vi "meTEC Control Software.vi"() -> ()   [LabVIEW 2019]
doc: "This is the vi discription of the Top Level VI"
uses:
  LV Source/[meerstetter engineering TE Cooling]/TypeDefs/meTEC_ID 50000_Live Enable.ctl
  LV Source/[meerstetter engineering TE Cooling]/TypeDefs/meTEC_ID 2000_Input Selection.ctl
  LV Source/[meerstetter engineering TE Cooling]/TypeDefs/meTEC_ID 50011_Object Target Temperature Source Selection.ctl
  LV Source/[meerstetter engineering TE Cooling]/TypeDefs/meTEC_ID 104_Device Status.ctl
  LV Source/[meerstetter engineering TE Cooling]/TypeDefs/meTEC_ID 1200_Temperature is Stable.ctl
  LV Source/Type Definitions/Main Loop Queue Data.ctl
  LV Source/Type Definitions/Main Loop States.ctl
  LV Source/Variables/FGVs/Type Defs/FGV_Operations.ctl
  <vilib>/Utility/error.llb/DialogType.ctl
  LV Source/Variables/Globals/Global_Initialized.vi
  LV Source/Variables/Globals/Global_TEC Monitor Loop_Status.vi
  LV Source/Variables/Globals/Global_Quit.vi
panel:
  out "Control Suite Status":string
  in  "Tab Control_General":T1(tab)
  out "meTEC_Device Type":string caption="Device Type"
  out "meTEC_CH1_Device Status":T2=1 caption="Device Status" items=["Initializing", "Ready", "Run", "Error", "Bootloader", "Reset in Progress"]
  out "meTEC_CH1_Temperature Stability":T3=1 caption="Temperature Stabilty" items=["Temperature regulation is not active", "Is not stable", "Is stable"]
  out "meTEC_CH1_Object Temperature [°C]":dbl caption="Object Temperature [°C]" format="%.3f"
  out "meTEC_CH1_Sink Temperature [°C]":dbl caption="Sink Temperature [°C]" format="%.3f"
  out "meTEC_CH1_Act. Output Voltage [V]":dbl caption="Act. Output Voltage [V]" format="%.3f"
  out "meTEC_CH1_Act. Output Current [A]":dbl caption="Act. Output Current [A]" format="%.3f"
  out "meTEC_Hardware Version":string caption="Hardware Version"
  out "meTEC_Firmware Version":string caption="Firmware Version"
  out "meTEC_Serial No.":i32 caption="Serial No."
  out "meTEC_CH1_Error No.":i32 caption="Error No."
  out "meTEC_CH1_Error Instance":i32 caption="Error Instance"
  out "meTEC_CH1_Error Parameter":i32 caption="Error Parameter"
  out "meTEC_CH2_Temperature Stability":T3=1 caption="Temperature Stabilty" items=["Temperature regulation is not active", "Is not stable", "Is stable"]
  out "meTEC_CH2_Act. Output Current [A]":dbl caption="Act. Output Current [A]" format="%.3f"
  out "meTEC_CH2_Act. Output Voltage [V]":dbl caption="Act. Output Voltage [V]" format="%.3f"
  out "meTEC_CH2_Object Temperature [°C]":dbl caption="Object Temperature [°C]" format="%.3f"
  out "meTEC_CH2_Sink Temperature [°C]":dbl caption="Sink Temperature [°C]" format="%.3f"
  out "Monitor Chart_CH2":dbl[](graph)
  out "Monitor Chart_CH1":dbl[](graph)
  out "Loop Rate [ms]":u32 caption="Update Rate [ms]"
  in  "meTEC_Reset Device":bool caption="Reset Device"
  in  "meTEC_CH1_Live Enable (ID 50000)":T4 caption="Live Enable (ID 50000)" items=["Disabled (Reset State)", "Enabled"]
  in  "meTEC_CH1_Input Selection (ID 2000)":T5=2 caption="Input  Selection (ID 2000)" items=["Static Current / Voltage", "Live Current / Voltage", "Temperature Controller"]
  in  "meTEC_CH1_Object Target Temp. Source Selection (ID 50011)":T6 caption="Object Target Temperature Source Selection (ID 50011)" items=["Parameter ID 3000 (Reset State)", "Parameter ID 50012"]
  in  "meTEC_CH1_Object Target Temperature (ID 3000 / 50012) [°C]":dbl=23.0 caption="Object Target Temperature (ID 3000 / 50012) [°C]" min=-273.0 max=1000.0 step=0.001 format="%#.3f"
  in  "meTEC_CH1_Live Set Current (ID 50001) [A]":dbl caption="Live Set Current (ID 50001) [A]" min=-16.0 max=16.0 step=0.001 format="%#.3f"
  in  "meTEC_CH2_Object Target Temperature (ID 3000 / 50012) [°C]":dbl=23.0 caption="Object Target Temperature (ID 3000) [°C]" min=-273.0 max=1000.0 step=0.001 format="%#.3f"
  in  "meTEC_CH2_Live Set Current (ID 50001) [A]":dbl caption="Live Set Current (ID 50001) [A]" min=-16.0 max=16.0 step=0.001 format="%#.3f"
  in  "meTEC_CH1_Live Set Voltage (ID 50002) [V]":dbl caption="Live Set Voltage (ID 50002) [V]" min=0.0 max=30.0 step=0.001 format="%#.3f"
  in  "meTEC_CH2_Live Set Voltage (ID 50002) [V]":dbl caption="Live Set Voltage (ID 50002) [V]" min=0.0 max=30.0 step=0.001 format="%#.3f"
  in  "meTEC_CH2_Object Target Temp. Source Selection (ID 50011)":T6 caption="Object Target Temperature Source Selection (ID 50011)" items=["Parameter ID 3000 (Reset State)", "Parameter ID 50012"]
  in  "meTEC_CH2_Input Selection (ID 2000)":T5=2 caption="Input  Selection (ID 2000)" items=["Static Current / Voltage", "Live Current / Voltage", "Temperature Controller"]
  in  "meTEC_CH2_Live Enable (ID 50000)":T4 caption="Live Enable" items=["Disabled (Reset State)", "Enabled"]
  in  "meTEC_Initialize Device":bool caption="Initialize Device"
  in  "meTEC_Perform Test":bool caption="Execute Test"
  out "Error History Table":string[][](table) caption="Error History"
  in  "Filepath Error Log File":path=path "C:/Error Data"
  in  "Show Pop-Ups for Error Messages?":bool
  in  "meTEC_Error Test 1_ID100_Device Type":bool caption="Error Test"
  # "Channel 1"
  # "Channel 2"
  # "General"
  # "Channel 1"
  # "Channel 2"
  # "Please set \"CH1 Output Stage Enable\" to\n\"Live ON/OFF\" in meerstetter engineering\nservice software.\n\nAfter that you can switch the TE controller\nON / OFF by changing the \"Live Enable\"\nsetting in this LabVIEW example."
  # "Please set \"CH2 Output Stage Enable\" to\n\"Live ON/OFF\" in meerstetter engineering\nservice software.\n\nAfter that you can switch the TE controller\nON / OFF by changing the \"Live Enable\"\nsetting in this LabVIEW example."
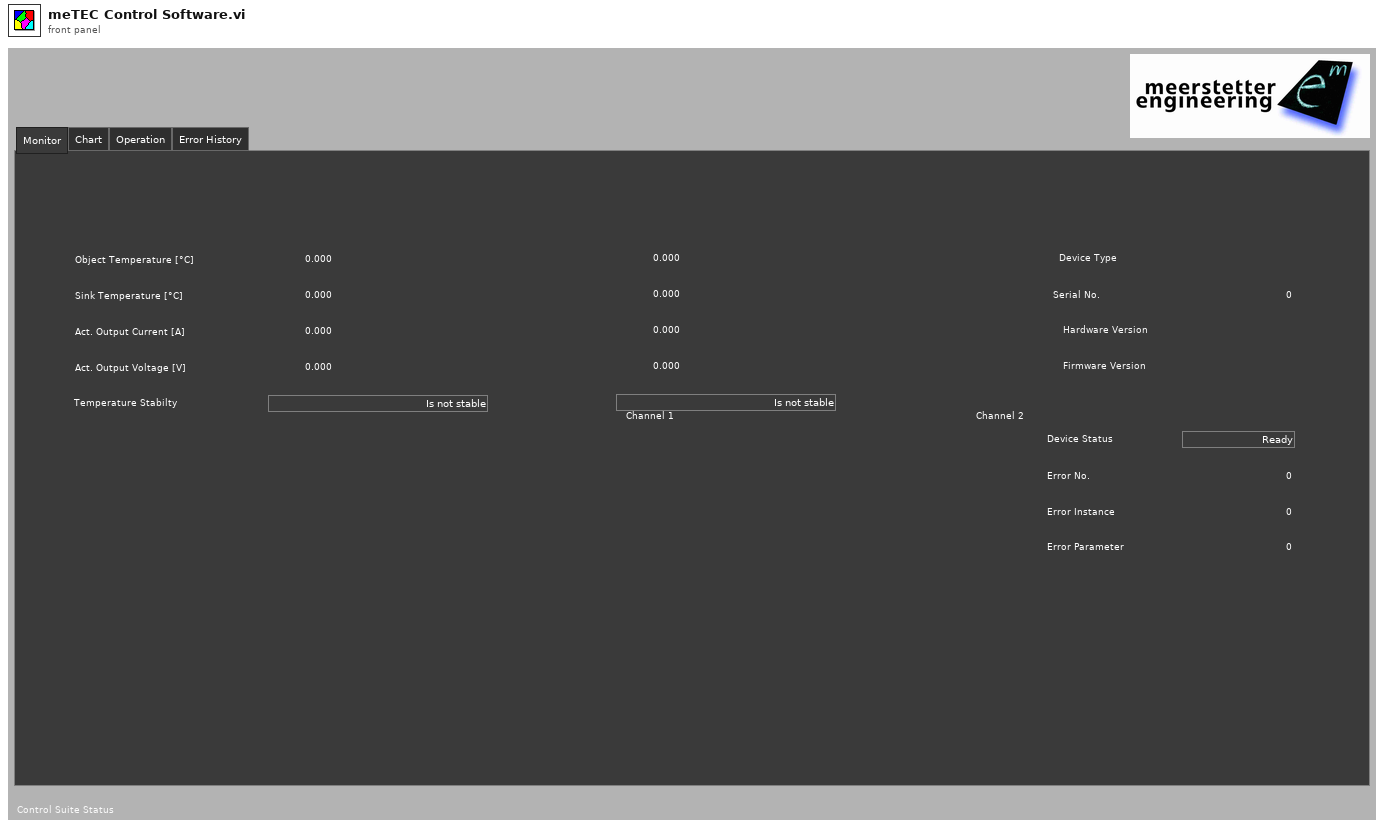
[diagram p1: front panel]
types:
  T1 = enum32{"Monitor", "Chart", "Operation", "Error History"}
  T2 = typedef "meTEC_ID 104_Device Status.ctl" = i32
  T3 = typedef "meTEC_ID 1200_Temperature is Stable.ctl" = i32
  T4 = typedef "meTEC_ID 50000_Live Enable.ctl" = i32
  T5 = typedef "meTEC_ID 2000_Input Selection.ctl" = i32
  T6 = typedef "meTEC_ID 50011_Object Target Temperature Source Selection.ctl" = i32
  T7 = typedef "Main Loop States.ctl" = enum16{"  -----  Core  -----  ", "Blank", "Idle", "Initialize", "Shutdown", "Error", "  ----- meerstetter TEC Functions -----  ", "TE Controller"}
  T8 = typedef "Main Loop Queue Data.ctl" = cluster{"Parameter":string, "Variant":variant, "Main Loop States":T7}
  T9 = enum32{"invalid app kind", "Development System", "Run Time System", "Student Edition", "Embedded LabVIEW", "Evaluation", "Custom"}
  T10 = typedef "FGV_Operations.ctl" = enum16{"Read", "Write"}
  T11 = typedef "FGV_TE Controller.ctl" = cluster{"SVs":cluster{"Unused":dbl}, "PVs":cluster{"FW & HW Versions":cluster{"Device Type [I32]":i32, "Device Type [String]":string, "Firmware Version [I32]":i32, "Firmware Version [String]":string, "Hardware Version [I32]":i32, "Hardware Version [String]":string, "Serial No.":i32}, "TEC Configuration":T12, "Object Target Temperature Source_CH1":u8, "Object Target Temperature Source_CH2":u8}, "Front Panel References":T13}
  T12 = typedef "meTEC_Configuration.ctl" = cluster{"VISA resource name":refnum<visa-resource-name>, "Device Address":u16}
  T13 = typedef "FGV_Front Panel References.ctl" = cluster{"Main Loop Queue":refnum<queue>, "meTEC_Device Type":refnum<vi>, "meTEC_Serial No.":refnum<vi>, "meTEC_Hardware Version":refnum<vi>, "meTEC_Firmware Version":refnum<vi>, "meTEC_CH1_Object Target Temperature (ID 3000 / 50012) [°C]":refnum<vi>, "meTEC_CH1_Live Set Current (ID 50001) [A]":refnum<vi>, "meTEC_CH1_Live Set Voltage (ID 50002) [V]":refnum<vi>, "meTEC_CH1_Live Enable (ID 50000)":refnum<vi>, "meTEC_CH1_Input Selection (ID 2000)":refnum<vi>, "meTEC_CH1_Object Target Temp. Source Sel. (ID 50011)":refnum<vi>, "meTEC_CH2_Object Target Temperature (ID 3000 / 50012) [°C]":refnum<vi>, "meTEC_CH2_Live Set Current (ID 50001) [A]":refnum<vi>, "meTEC_CH2_Live Set Voltage (ID 50002) [V]":refnum<vi>, "meTEC_CH2_Live Enable (ID 50000)":refnum<vi>, "meTEC_CH2_Input Selection (ID 2000)":refnum<vi>, "meTEC_CH2_Object Target Temp. Source Sel. (ID 50011)":refnum<vi>, "meTEC_CH2_Object Temperature [°C]":refnum<vi>, "meTEC_CH2_Sink Temperature [°C]":refnum<vi>, "meTEC_CH2_Act. Output Current [A]":refnum<vi>, "meTEC_CH2_Act. Output Voltage [V]":refnum<vi>, "meTEC_CH2_Temperature Stability":refnum<vi>, "Monitor Chart_CH2":refnum<vi>, "meTEC_Initialize Device":refnum<vi>}
  T14 = typedef "DialogType.ctl" = u16
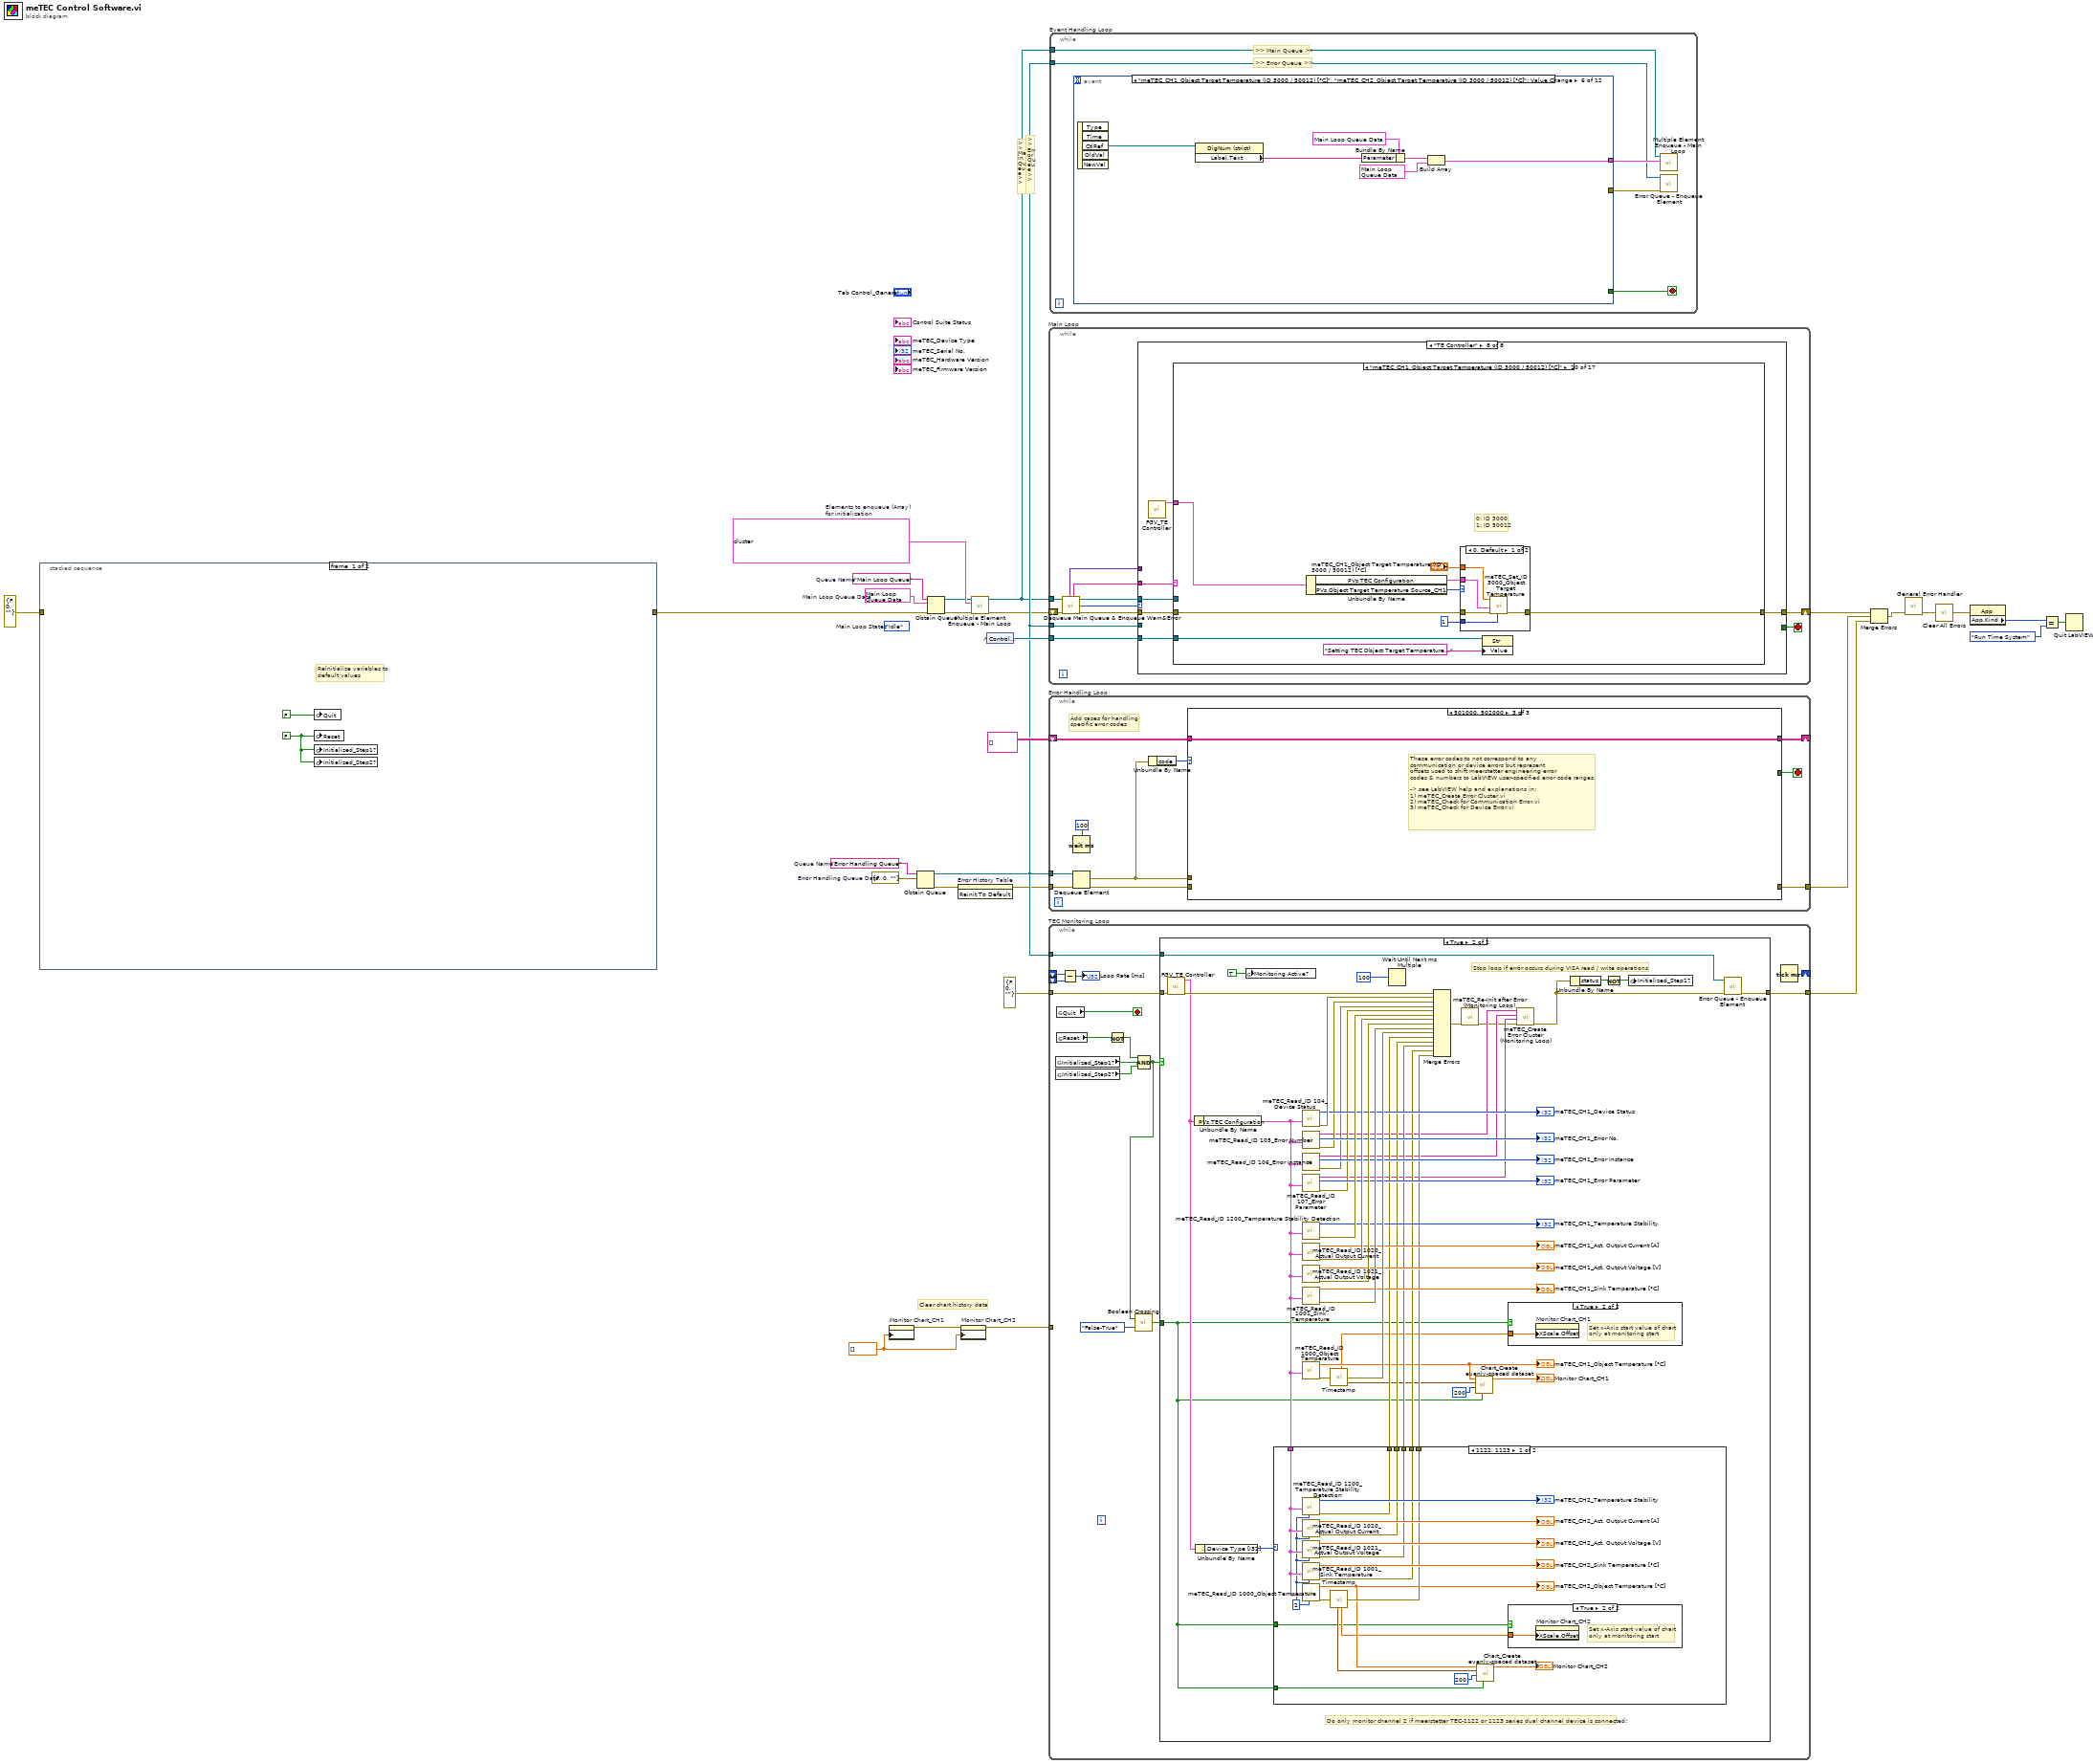
[diagram p0: block diagram]
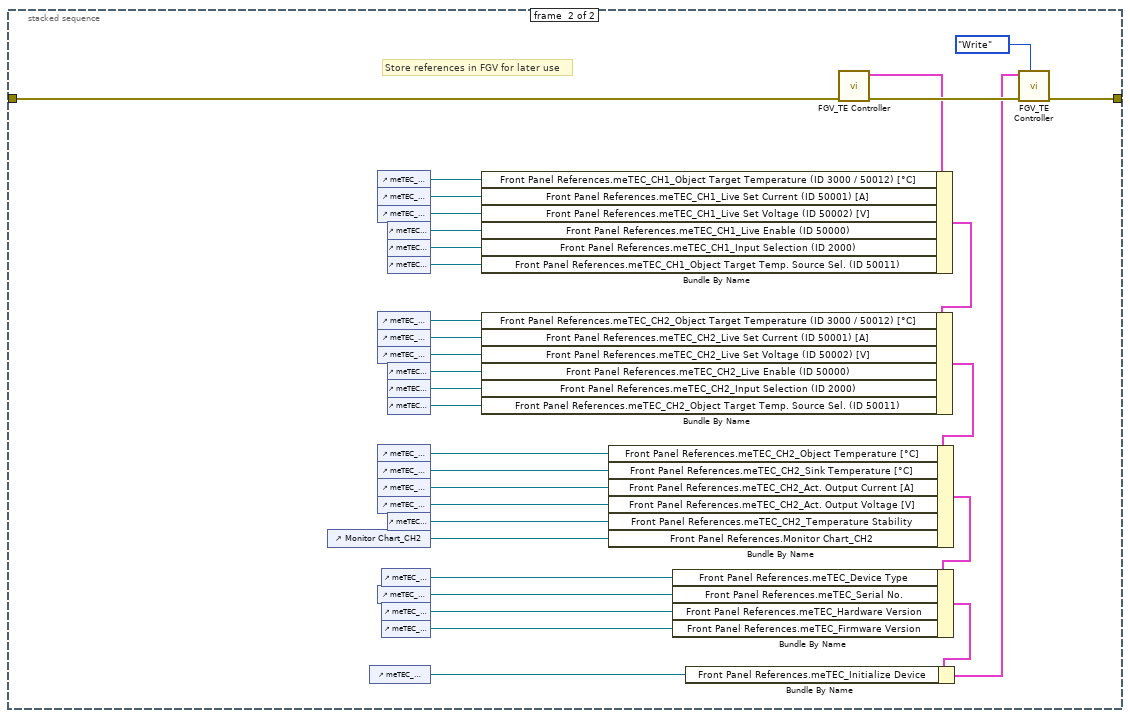
[diagram p2: hidden frame]
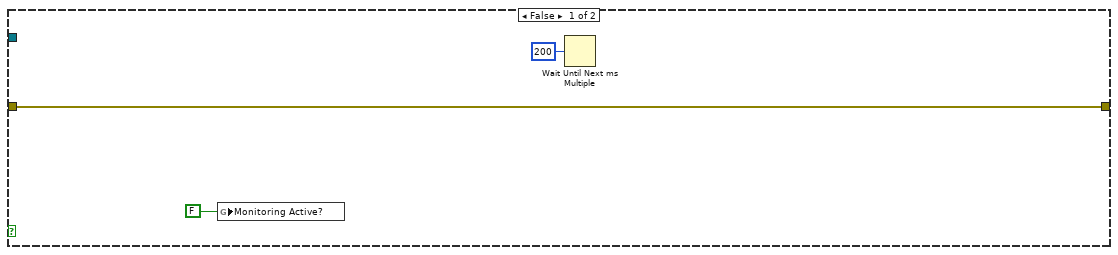
[diagram p3: hidden frame]
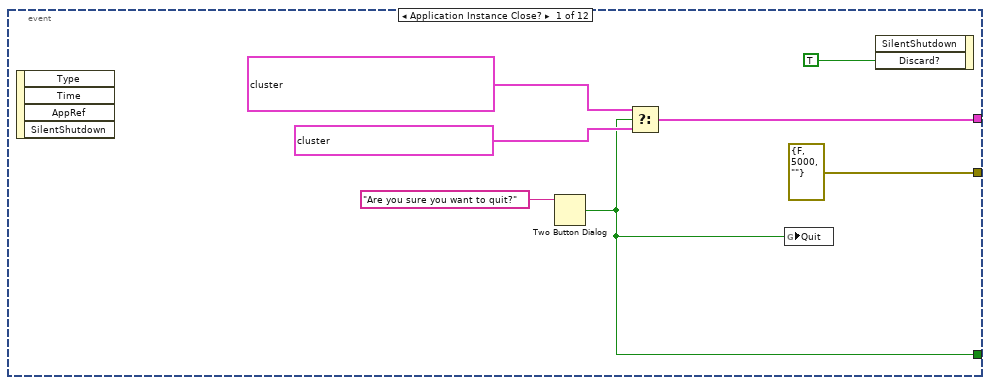
[diagram p7: hidden frame]
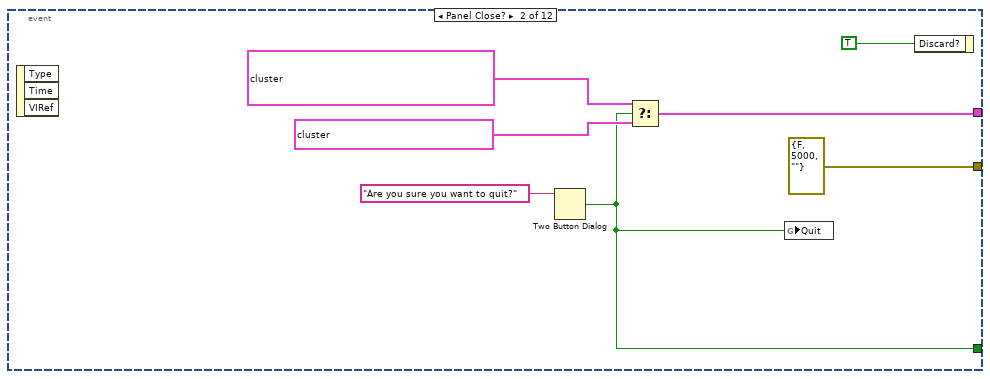
[diagram p8: hidden frame]
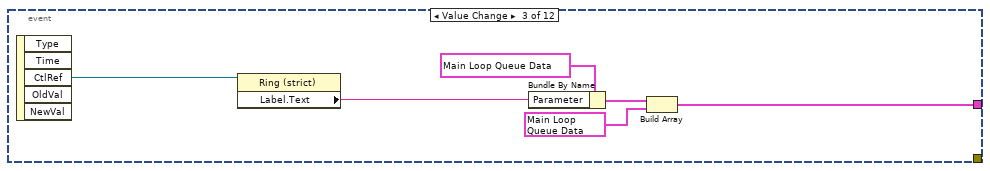
[diagram p9: hidden frame]
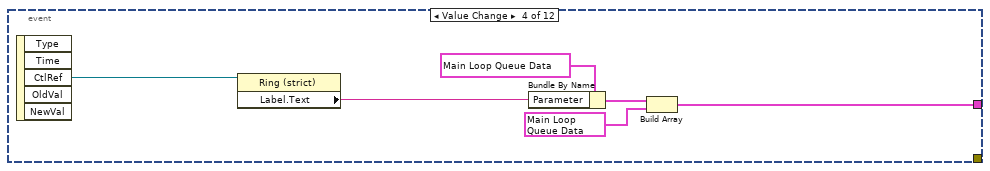
[diagram p10: hidden frame]
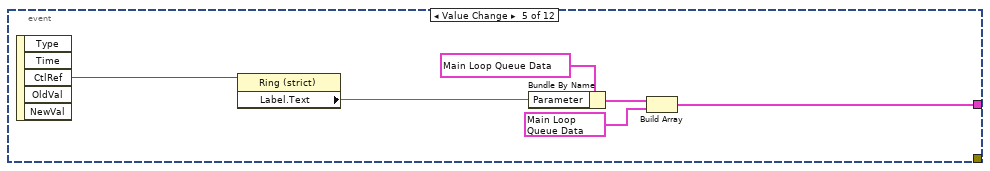
[diagram p11: hidden frame]
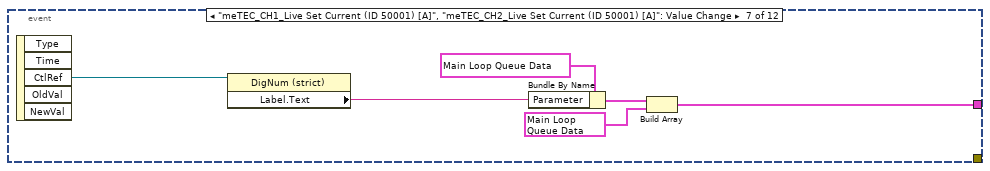
[diagram p12: hidden frame]
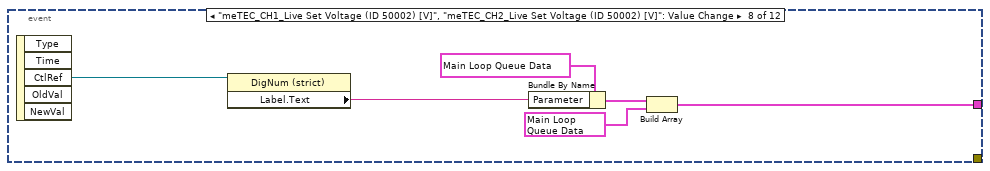
[diagram p13: hidden frame]
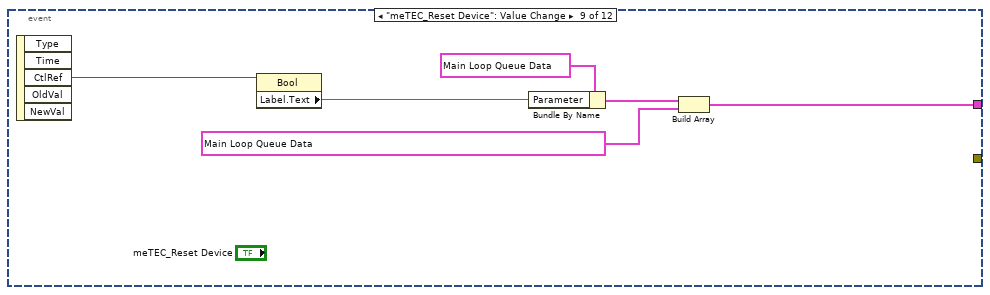
[diagram p14: hidden frame]
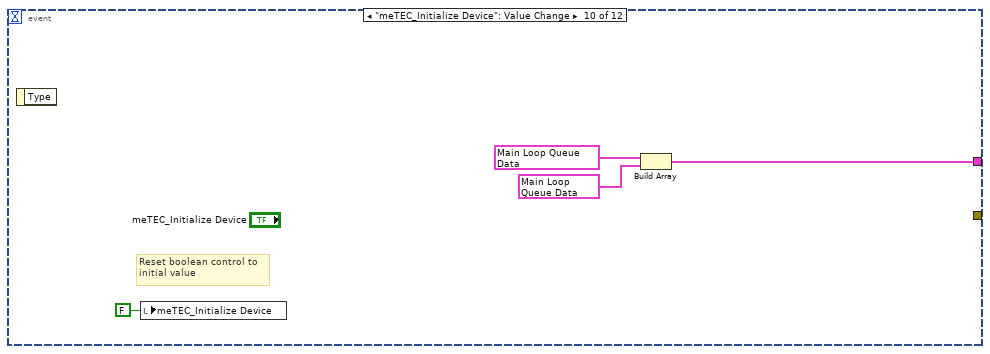
[diagram p15: hidden frame]
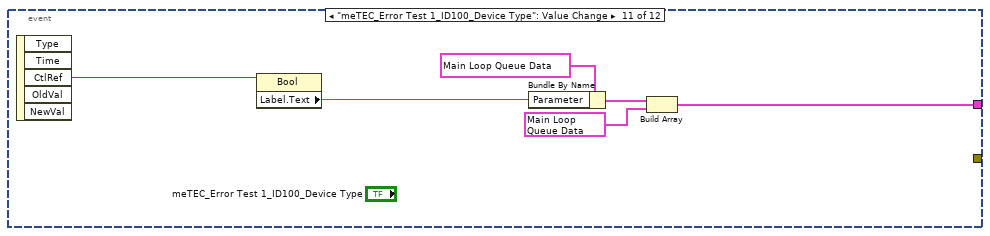
[diagram p16: hidden frame]
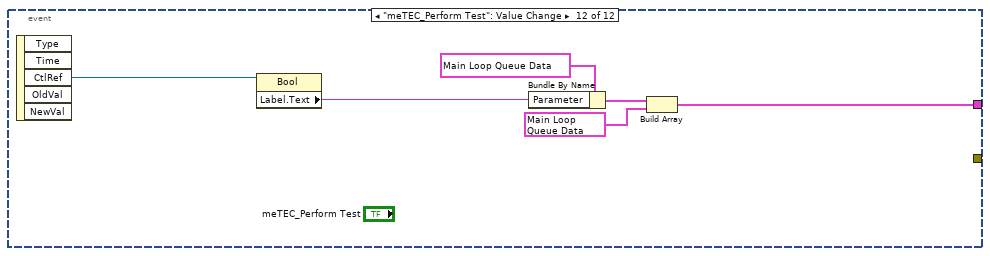
[diagram p17: hidden frame]
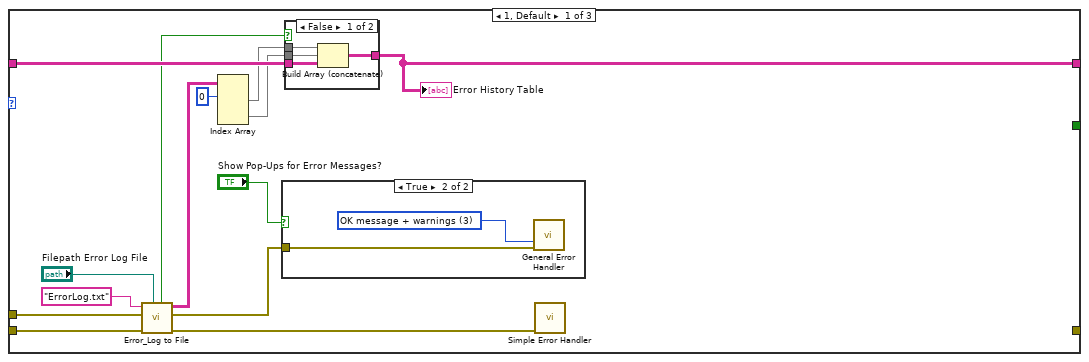
[diagram p18: hidden frame]
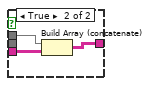
[diagram p19: hidden frame]
diagram:
  w7 = dbl[] [] ("History Data")
  (unwired) Main_Loop_States."Idle"  # Main Loop States
  w19 = T8 {"Parameter"="", "Variant"=variant, "Main Loop States"=enum."Idle"}  # Main Loop Queue Data
  w24 = errorcluster {"status"=FALSE, "code"=0, "source"=""}  # Error Handling Queue Data
  w25 = "Error Handling Queue"  # Queue Name
  w26 = "Main Loop Queue"  # Queue Name
  w18 = T8[] [{"Parameter"="", "Variant"=variant, "Main Loop States"=enum."Initialize"}, {"Parameter"="", "Variant"=variant, "Main Loop States"=enum."Idle"}]  # Elements to enqueue (Array) for initialization
  # "Clear chart history data"
  # ">> Error Queue >>"
  # ">> Main Queue >>"
  n1 = stacked-sequence {
    tunnel: [_ w63] -> w11
    tunnel: errorcluster {"status"=FALSE, "code"=0, "source"=""} ("error out") -> [_ w64]
    frame #0 {
      w31 = FALSE ("Error")
      # "Reinitialize variables to\ndefault values"
      n2 = global write "Global_Quit.vi" "Quit"(FALSE ("Quit")) -> ()
      n3 = global write "Global_TEC Monitor Loop_Status.vi" "Reset"(w31) -> ()
      n4 = global write "Global_Initialized.vi" "Initialized_Step1?"(w31) -> ()
      n5 = global write "Global_Initialized.vi" "Initialized_Step2?"(w31) -> ()
    }
    frame #1 {
      # "Store references in FGV for later use"
      n6 = control-ref of="Monitor Chart_CH2"() -> (w43:refnum<vi>)
      n7 = control-ref of="meTEC_Initialize Device"() -> (w38:refnum<vi>)
      n8 = control-ref of="meTEC_CH1_Object Target Temperature (ID 3000 / 50012) [°C]"() -> (w46:refnum<vi>)
      n9 = control-ref of="meTEC_CH1_Live Set Current (ID 50001) [A]"() -> (w44:refnum<vi>)
      n10 = control-ref of="meTEC_CH1_Live Set Voltage (ID 50002) [V]"() -> (w45:refnum<vi>)
      n11 = control-ref of="meTEC_CH2_Object Target Temperature (ID 3000 / 50012) [°C]"() -> (w60:refnum<vi>)
      n12 = control-ref of="meTEC_CH2_Live Set Current (ID 50001) [A]"() -> (w55:refnum<vi>)
      n13 = control-ref of="meTEC_CH2_Live Set Voltage (ID 50002) [V]"() -> (w56:refnum<vi>)
      n14 = control-ref of="meTEC_CH2_Object Temperature [°C]"() -> (w53:refnum<vi>)
      n15 = control-ref of="meTEC_CH2_Sink Temperature [°C]"() -> (w49:refnum<vi>)
      n16 = control-ref of="meTEC_CH2_Act. Output Current [A]"() -> (w50:refnum<vi>)
      n17 = control-ref of="meTEC_CH2_Act. Output Voltage [V]"() -> (w51:refnum<vi>)
      n18 = control-ref of="meTEC_Serial No."() -> (w34:refnum<vi>)
      n19 = control-ref of="meTEC_Device Type"() -> (w35:refnum<vi>)
      n20 = control-ref of="meTEC_Hardware Version"() -> (w33:refnum<vi>)
      n21 = control-ref of="meTEC_Firmware Version"() -> (w32:refnum<vi>)
      n22 = control-ref of="meTEC_CH1_Live Enable (ID 50000)"() -> (w41:refnum<vi>)
      n23 = control-ref of="meTEC_CH1_Input Selection (ID 2000)"() -> (w40:refnum<vi>)
      n24 = control-ref of="meTEC_CH1_Object Target Temp. Source Selection (ID 50011)"() -> (w39:refnum<vi>)
      n25 = control-ref of="meTEC_CH2_Live Enable (ID 50000)"() -> (w57:refnum<vi>)
      n26 = control-ref of="meTEC_CH2_Input Selection (ID 2000)"() -> (w58:refnum<vi>)
      n27 = control-ref of="meTEC_CH2_Object Target Temp. Source Selection (ID 50011)"() -> (w59:refnum<vi>)
      n28 = control-ref of="meTEC_CH2_Temperature Stability"() -> (w52:refnum<vi>)
      n29 = call "FGV_TE Controller.vi"("error in (no error)"=w64) -> ("error out"=w62:errorcluster, "FGV_TEC_OUT"=w48:T11)  [unwired: 9 in]
      n30 = Bundle By Name(cluster=w48, "Front Panel References.meTEC_CH1_Object Target Temperature (ID 3000 / 50012) [°C]"=w46, "Front Panel References.meTEC_CH1_Live Set Current (ID 50001) [A]"=w44, "Front Panel References.meTEC_CH1_Live Set Voltage (ID 50002) [V]"=w45, "Front Panel References.meTEC_CH1_Live Enable (ID 50000)"=w41, "Front Panel References.meTEC_CH1_Input Selection (ID 2000)"=w40, "Front Panel References.meTEC_CH1_Object Target Temp. Source Sel. (ID 50011)"=w39) -> (w47:T11)
      n31 = Bundle By Name(cluster=w47, "Front Panel References.meTEC_CH2_Object Target Temperature (ID 3000 / 50012) [°C]"=w60, "Front Panel References.meTEC_CH2_Live Set Current (ID 50001) [A]"=w55, "Front Panel References.meTEC_CH2_Live Set Voltage (ID 50002) [V]"=w56, "Front Panel References.meTEC_CH2_Live Enable (ID 50000)"=w57, "Front Panel References.meTEC_CH2_Input Selection (ID 2000)"=w58, "Front Panel References.meTEC_CH2_Object Target Temp. Source Sel. (ID 50011)"=w59) -> (w54:T11)
      n32 = Bundle By Name(cluster=w54, "Front Panel References.meTEC_CH2_Object Temperature [°C]"=w53, "Front Panel References.meTEC_CH2_Sink Temperature [°C]"=w49, "Front Panel References.meTEC_CH2_Act. Output Current [A]"=w50, "Front Panel References.meTEC_CH2_Act. Output Voltage [V]"=w51, "Front Panel References.meTEC_CH2_Temperature Stability"=w52, "Front Panel References.Monitor Chart_CH2"=w43) -> (w37:T11)
      n33 = Bundle By Name(cluster=w37, "Front Panel References.meTEC_Device Type"=w35, "Front Panel References.meTEC_Serial No."=w34, "Front Panel References.meTEC_Hardware Version"=w33, "Front Panel References.meTEC_Firmware Version"=w32) -> (w36:T11)
      n34 = Bundle By Name(cluster=w36, "Front Panel References.meTEC_Initialize Device"=w38) -> (w42:T11)
      n35 = call "FGV_TE Controller.vi"("Operation (Read)"=FGV_Operations."Write", "error in (no error)"=w62, "FGV_TEC_IN"=w42) -> ("error out"=w63:errorcluster)  [unwired: 7 in, 1 out]
    }
  }
  n36 = property on="Monitor Chart_CH1" class="WFChart (strict)"("History Data"=w7) -> (error out=w9:errorcluster)  [unwired: 2 in, 1 out]
  n37 = Obtain Queue(name (unnamed)=w25, element data type=w24) -> (queue out=w5:refnum<queue>, error out=w4:errorcluster)  [unwired: 3 in, 1 out]
  n38 = Obtain Queue(name (unnamed)=w26, element data type=w19, error in (no error)=w11) -> (queue out=w17:refnum<queue>, error out=w12:errorcluster)  [unwired: 2 in, 1 out]
  n39 = invoke on="Error History Table" class="Tbl (strict)" method="Reinit To Default"(error in=w4) -> (error out=w3:errorcluster)  [unwired: 2 in, 2 out]
  n40 = property on="Monitor Chart_CH2" class="WFChart (strict)"(error in=w9, "History Data"=w7) -> (error out=w8:errorcluster)  [unwired: 1 in, 1 out]
  n41 = call "Multiple Element Enqueue - Main Loop.vi"("error in (no error)"=w12, "Elements to enqueue (Array)"=w18, "Queue In"=w17) -> ("error out"=w1:errorcluster, "QueueOut"=w2:refnum<queue>)  [unwired: 7 in]
  n42 = control-ref of="Control Suite Status"() -> (w15:refnum<vi>)
  n43 = while "Error Handling Loop" {
    tunnel: w5 -> [w74]
    shift-right: [w69] -> _
    shift-left: string[][] [] -> [w68]
    tunnel: w3 -> [w73]
    tunnel: [w72] -> w22
    stop <- w70 stop-if-true
    # "Add cases for handling\nspecific error codes"
    n44 = Wait (ms)(milliseconds to wait=u32 100) -> ()  [unwired: 1 out]
    n45 = Dequeue Element(queue=w74, error in (no error)=w73) -> (element=w66:errorcluster, error out=w65:errorcluster)  [unwired: 1 in, 2 out]
    n46 = Unbundle By Name(w66) -> ("code"=w67:i32)
    n47 = case shown="501000, 502000" w67 {
      tunnel: [_ w98 _] -> w72
      tunnel: w66 -> [w81 _ _]
      tunnel: [_ TRUE _] -> w70
      tunnel: [w88 w100 w101] -> w69
      tunnel: w68 -> [w87 w100 w101]
      tunnel: w65 -> [w84 w98 _]
      frame 1, Default {
        n48 = call "Error_Log to File.vi"("Error Log Filepath"="Filepath Error Log File", "error in (no error)"=w84, "Error Data_IN"=w81, "Error Log Filename"="ErrorLog.txt" ("Rel. Path\\Filename")) -> ("error out"=w86:errorcluster, "Error Data_OUT"=w80:errorcluster, "Error Data (2D String Array)"=w77:string[][], "Call chain empty?"=w75:bool)  [unwired: 4 in]
        n49 = Index Array(array=w77, index (row) #1=0 ("index (row)")) -> (element #1=w78:string[], element #2=w76:string[])  [unwired: 3 in]
        n50 = case shown="True" "Show Pop-Ups for Error Messages?" {
          tunnel: w80 -> [_ w97]
          frame False {
          }
          frame True {
            w96 = T14 3 items=["no dialog", "OK message", "continue or stop message", "OK message + warnings", "continue/stop + warnings"] ("type of dialog (OK msg:1)")
            n51 = call <vilib>:"General Error Handler.vi"("type of dialog (OK msg:1)"=w96, "error in (no error)"=w97) -> ()  [unwired: 9 in, 5 out]
          }
        }
        n52 = case shown="False" w75 {
          tunnel: [w92 w95] -> w88
          tunnel: w87 -> [w91 w94]
          tunnel: w78 -> [w90 w93]
          tunnel: w76 -> [w89 _]
          frame False {
            n53 = Build Array (concatenate)(w90, w89, w91) -> (w92:string[][])
          }
          frame True {
            n54 = Build Array (concatenate)(w93, w94) -> (w95:string[][])
          }
        }
        "Error History Table" <- w88
        n55 = call <vilib>:"Simple Error Handler.vi"("error in (no error)"=w86) -> ()  [unwired: 4 in, 5 out]
      }
      frame 5000 {
        # "Application quit by user request"
      }
      frame 501000, 502000 {
        # "These error codes to not correspond to any\ncommunication or device errors but represent\noffsets used to shift meerstetter engineering error\ncodes & numbers to LabVIEW user-specified error code ranges.\n\n-> see LabVIEW help and explanations in:\n1) meTEC_Create Error Cluster.vi\n2) meTEC_Check for Communication Error.vi\n3) meTEC_Check for Device Error.vi"
      }
    }
  }
  n56 = while "TEC Monitoring Loop" {
    tunnel: errorcluster {"status"=FALSE, "code"=0, "source"=""} ("error in") -> [w115]
    tunnel: w5 -> [w116]
    tunnel: [w114] -> w13
    shift-right: [w113] -> _
    shift-left: _ -> [w112]
    shift-left: _ -> [w111]
    tunnel: w8 -> [_]
    stop <- w103 stop-if-true
    n57 = global read "Global_Initialized.vi" "Initialized_Step1?"() -> (w106:bool)
    n58 = global read "Global_Initialized.vi" "Initialized_Step2?"() -> (w107:bool)
    n59 = global read "Global_Quit.vi" "Quit"() -> (w103:bool)
    n60 = global read "Global_TEC Monitor Loop_Status.vi" "Reset"() -> (w109:bool)
    n61 = Subtract(x=w112, y=w111) -> (x-y=→"Loop Rate [ms]":u32)
    n62 = Not(x=w109) -> (.not. x?=w108:bool)
    n63 = Compound Arithmetic op=AND(w108, w106, w107) -> (w105:bool)
    n64 = call "Boolean Crossing.vi"("Direction"=enum8{"Either", "False-True", "True-False"}."False-True", "Input"=w105) -> ("Crossing"=w104:bool)  [unwired: 1 in]
    n65 = case shown="True" w105 {
      tunnel: w115 -> [w119 w162]
      tunnel: [w119 w164] -> w114
      tunnel: w116 -> [_ w165]
      tunnel: w104 -> [_ w128]
      frame False {
        n66 = global write "Global_TEC Monitor Loop_Status.vi" "Monitoring Active?"(FALSE ("Error")) -> ()
        n67 = Wait Until Next ms Multiple(millisecond multiple=u32 200) -> ()  [unwired: 1 out]
      }
      frame True {
        # "Do only monitor channel 2 if meerstetter TEC-1122 or 1123 series dual channel device is connected!"
        # "Stop loop if error occurs during VISA read / write operations"
        n68 = call "FGV_TE Controller.vi"("error in (no error)"=w162) -> ("error out"=w161:errorcluster, "FGV_TEC_OUT"=w137:T11)  [unwired: 9 in]
        n69 = Unbundle By Name(w137) -> ("PVs.TEC Configuration"=w135:T12)
        n70 = Unbundle By Name(w137) -> ("PVs.FW & HW Versions.Device Type [I32]"=w136:i32)
        n71 = global write "Global_TEC Monitor Loop_Status.vi" "Monitoring Active?"(TRUE ("Error")) -> ()
        n72 = case shown="1122, 1123" w136 {
          tunnel: w135 -> [w180 _]
          tunnel: [w179 _] -> w142
          tunnel: [w178 _] -> w141
          tunnel: [w177 _] -> w140
          tunnel: [w176 _] -> w139
          tunnel: [w175 _] -> w138
          tunnel: w128 -> [w171 _]
          tunnel: w128 -> [w167 _]
          frame 1122, 1123 {
            w174 = u8 2 ("Instance (1)")
            n73 = call "meTEC_Read_ID 1200_Temperature Stability Detection.vi"("Instance (1)"=w174, "TEC Configuration_IN"=w180) -> ("error out"=w179:errorcluster, "Temperature is Stable? [I32)] (ID 1200)"=→"meTEC_CH2_Temperature Stability":i32)  [unwired: 6 in, 2 out]
            n74 = call "meTEC_Read_ID 1020_Actual Output Current.vi"("Instance (1)"=w174, "TEC Configuration_IN"=w180) -> ("error out"=w178:errorcluster, "Act. Output Current [A] (ID 1020)"=→"meTEC_CH2_Act. Output Current [A]":dbl)  [unwired: 7 in, 1 out]
            n75 = call "meTEC_Read_ID 1021_Actual Output Voltage.vi"("Instance (1)"=w174, "TEC Configuration_IN"=w180) -> ("error out"=w177:errorcluster, "Act. Output Voltage [A] (ID 1021)"=→"meTEC_CH2_Act. Output Voltage [V]":dbl)  [unwired: 7 in, 1 out]
            n76 = call "meTEC_Read_ID 1001_Sink Temperature.vi"("Instance (1)"=w174, "TEC Configuration_IN"=w180) -> ("error out"=w176:errorcluster, "Sink Temperature [°C] (ID 1001)"=→"meTEC_CH2_Sink Temperature [°C]":dbl)  [unwired: 7 in, 1 out]
            n77 = call "meTEC_Read_ID 1000_Object Temperature.vi"("Instance (1)"=w174, "TEC Configuration_IN"=w180) -> ("error out"=w181:errorcluster, "Object Temperature [°C] (ID 1000)"=w172:dbl)  [unwired: 7 in, 1 out]
            "meTEC_CH2_Object Temperature [°C]" <- w172
            n78 = call "Timestamp.vi"("error in (no error)"=w181) -> ("current time (time stamp)"=w173:timestamp, "current time (sec)"=w168:dbl, "error out"=w175:errorcluster)
            n79 = call "Chart_Create evenly-spaced dataset.vi"("Initialize?"=w171, "X-Axis Time Interval (100) [ms]"=200, "X (Time Stamp)"=w173, "Y (DBL)"=w172) -> ("Y (Interpolated array)"=→"Monitor Chart_CH2":dbl[])  [unwired: 6 in, 1 out]
            n80 = case shown="True" w167 {
              tunnel: w168 -> [_ w186]
              frame False {
              }
              frame True {
                # "Set x-Axis start value of chart\nonly at monitoring start"
                n81 = property on="Monitor Chart_CH2" class="WFChart (strict)"("XScale.Offset"=w186) -> ()  [unwired: 2 in, 2 out]
              }
            }
          }
          frame 1089..1091, Default {
          }
        }
        n82 = call "meTEC_Read_ID 104_Device Status.vi"("TEC Configuration_IN"=w135) -> ("error out"=w150:errorcluster, "Device Status (ID 104) [I32]"=→"meTEC_CH1_Device Status":i32)  [unwired: 8 in, 1 out]
        n83 = call "meTEC_Read_ID 105_Error Number.vi"("TEC Configuration_IN"=w135) -> ("error out"=w145:errorcluster, "Error Number (ID 105) [I32]"=→"meTEC_CH1_Error No.":i32, "Error Number (ID 105) [String]"=w123:string)  [unwired: 7 in, 1 out]
        n84 = call "meTEC_Read_ID 106_Error Instance.vi"("TEC Configuration_IN"=w135) -> ("error out"=w144:errorcluster, "Error Instance (ID 106) [I32]"=→"meTEC_CH1_Error Instance":i32, "Error Instance (ID 106) [String]"=w124:string)  [unwired: 7 in, 1 out]
        n85 = call "meTEC_Read_ID 107_Error Parameter.vi"("TEC Configuration_IN"=w135) -> ("error out"=w143:errorcluster, "Error Parameter (ID 107) [I32]"=→"meTEC_CH1_Error Parameter":i32, "Error Parameter (ID 107) [String]"=w125:string)  [unwired: 7 in, 1 out]
        n86 = call "meTEC_Read_ID 1200_Temperature Stability Detection.vi"("TEC Configuration_IN"=w135) -> ("error out"=w160:errorcluster, "Temperature is Stable? [I32)] (ID 1200)"=→"meTEC_CH1_Temperature Stability":i32)  [unwired: 7 in, 2 out]
        n87 = call "meTEC_Read_ID 1020_Actual Output Current.vi"("TEC Configuration_IN"=w135) -> ("error out"=w159:errorcluster, "Act. Output Current [A] (ID 1020)"=→"meTEC_CH1_Act. Output Current [A]":dbl)  [unwired: 8 in, 1 out]
        n88 = call "meTEC_Read_ID 1021_Actual Output Voltage.vi"("TEC Configuration_IN"=w135) -> ("error out"=w158:errorcluster, "Act. Output Voltage [A] (ID 1021)"=→"meTEC_CH1_Act. Output Voltage [V]":dbl)  [unwired: 8 in, 1 out]
        n89 = call "meTEC_Read_ID 1001_Sink Temperature.vi"("TEC Configuration_IN"=w135) -> ("error out"=w157:errorcluster, "Sink Temperature [°C] (ID 1001)"=→"meTEC_CH1_Sink Temperature [°C]":dbl)  [unwired: 8 in, 1 out]
        n90 = call "meTEC_Read_ID 1000_Object Temperature.vi"("TEC Configuration_IN"=w135) -> ("error out"=w156:errorcluster, "Object Temperature [°C] (ID 1000)"=w134:dbl)  [unwired: 8 in, 1 out]
        "meTEC_CH1_Object Temperature [°C]" <- w134
        n91 = call "Timestamp.vi"("error in (no error)"=w156) -> ("current time (time stamp)"=w133:timestamp, "current time (sec)"=w132:dbl, "error out"=w155:errorcluster)
        n92 = Wait Until Next ms Multiple(millisecond multiple=u32 100 ("TEC_Loop wait time [ms]")) -> ()  [unwired: 1 out]
        n93 = Merge Errors(w161, w150, w145, w144, w143, w160, w159, w158, w157, w155, w142, w141, w140, w139, w138) -> (w127:errorcluster)
        n94 = call "meTEC_Re-Init after Error (Monitoring Loop).vi"("error in (no error)"=w127) -> ("error out"=w120:errorcluster)  [unwired: 10 in]
        n95 = call "Chart_Create evenly-spaced dataset.vi"("Initialize?"=w128, "X-Axis Time Interval (100) [ms]"=200, "X (Time Stamp)"=w133, "Y (DBL)"=w134) -> ("Y (Interpolated array)"=→"Monitor Chart_CH1":dbl[])  [unwired: 6 in, 1 out]
        n96 = case shown="True" w128 {
          tunnel: w132 -> [_ w166]
          frame False {
          }
          frame True {
            # "Set x-Axis start value of chart\nonly at monitoring start"
            n97 = property on="Monitor Chart_CH1" class="WFChart (strict)"("XScale.Offset"=w166) -> ()  [unwired: 2 in, 2 out]
          }
        }
        n98 = call "meTEC_Create Error Cluster (Monitoring Loop).vi"("error in (no error)"=w120, "Error Parameter"=w125, "Error Instance"=w124, "Error Number"=w123) -> ("error out"=w126:errorcluster)  [unwired: 7 in]
        n99 = Unbundle By Name(w126) -> ("status"=w122:bool)
        n100 = Not(x=w122) -> (.not. x?=w121:bool)
        n101 = global write "Global_Initialized.vi" "Initialized_Step1?"(w121) -> ()
        n102 = call "Error Queue - Enqueue Element.vi"("error in (no error)"=w126, "Error Queue IN"=w165) -> ("error out"=w164:errorcluster)  [unwired: 9 in]
      }
    }
    n103 = Tick Count (ms)() -> (millisecond timer value=w113:u32)
  }
  n104 = while "Main Loop" {
    tunnel: w2 -> [w194]
    shift-right: [w196] -> w23
    shift-left: w1 -> [w193]
    tunnel: w5 -> [w195]
    tunnel: w15 -> [w187]
    stop <- w197 stop-if-true
    n105 = call "Dequeue Main Queue & Enqueue Warn&Error.vi"("error in (no error)"=w193, "Queue In"=w194) -> ("error out (no error)"=w192:errorcluster, "Main Loop State"=w190:T7, "Queue Out"=w191:refnum<queue>, "Parameter"=w189:string, "Variant"=w188:variant)  [unwired: 5 in]
    n106 = case shown="\"TE Controller\"" w190 {
      tunnel: [_ _ _ _ TRUE _ _ _] -> w197
      tunnel: w192 -> [w198 w200 _ w212 w213 w226 w235 w241]
      tunnel: [w198 w200 _ w209 w217 w222 w235 w240] -> w196
      tunnel: w195 -> [_ _ _ w211 w216 w227 _ _]
      tunnel: w191 -> [_ _ _ _ _ w224 _ w236]
      tunnel: w189 -> [_ _ _ _ _ _ _ w238]
      tunnel: w188 -> [_ _ _ _ _ _ _ _]
      tunnel: w187 -> [_ w201 w206 w210 w214 _ _ w239]
      frame "  -----  Core  -----  " {
      }
      frame "Blank" {
        n107 = property class="Str"(reference=w201, "Value"="Process Description...") -> ()  [unwired: 1 in, 2 out]
      }
      frame "Idle", Default {
        n108 = global read "Global_Initialized.vi" "Initialized_Step1?"() -> (w204:bool)
        n109 = Select(t="Idle" ("Value"), s=w204, f="No TE Controller connected!" ("Value")) -> (s? t:f=w205:string)
        n110 = case shown="True" w204 {
          frame False {
            # "In case initialization failed, e.g. because no TEC was yet \nconnected or energized, the initialization routine is triggered\nagain after a specified wait time."
            n111 = flat-sequence {
              frame #0 {
                n112 = Wait (ms)(milliseconds to wait=u32 2000) -> ()  [unwired: 1 out]
              }
              frame #1 {
                n113 = property on="meTEC_Initialize Device" class="Bool (strict)"("Val(Sgnl)"=TRUE) -> ()  [unwired: 2 in, 2 out]
              }
            }
          }
          frame True {
          }
        }
        n114 = property class="Str"(reference=w206, "Value"=w205) -> ()  [unwired: 1 in, 2 out]
      }
      frame "Initialize" {
        # "Initialize TE Controller"
        n115 = call "Initialize System.vi"("System Status"=w210, "Error Queue"=w211, "error in (no error)"=w212) -> ("error out"=w209:errorcluster)  [unwired: 8 in]
      }
      frame "Shutdown" {
        n116 = call "Shutdown System.vi"("System Status"=w214, "Error Queue"=w216, "error in (no error)"=w213) -> ("error out"=w217:errorcluster)  [unwired: 8 in]
      }
      frame "Error" {
        (unwired) i32[] []
        # "List all error codes in this array which require a queue flush"
        n117 = Unbundle By Name(w226) -> ("code"=w225:i32, "status"=w219:bool)
        n118 = Enqueue Element(queue=w227, element=w226) -> (error out=w223:errorcluster)  [unwired: 2 in, 2 out]
        n119 = Equal?(x=-8000, y=w225) -> (x = y?=w220:bool)
        n120 = And(x=w220, y=w219) -> (x .and. y?=w218:bool)
        n121 = case shown="True" w218 {
          tunnel: w224 -> [_ w234]
          tunnel: w223 -> [w228 w233]
          tunnel: [w228 w231] -> w222
          frame False {
          }
          frame True {
            # "Execute specified\nstates in case of error"
            # "Flush Queue"
            n122 = Flush Queue(queue=w234, error in (no error)=w233) -> (queue out=w230:refnum<queue>, error out=w232:errorcluster)  [unwired: 1 out]
            n123 = call "Multiple Element Enqueue - Main Loop.vi"("error in (no error)"=w232, "Elements to enqueue (Array)"=T8[] [], "Queue In"=w230) -> ("error out"=w231:errorcluster)  [unwired: 7 in, 1 out]
          }
        }
      }
      frame "  ----- meerstetter TEC Functions -----  " {
      }
      frame "TE Controller" {
        n124 = call "FGV_TE Controller.vi"() -> ("FGV_TEC_OUT"=w237:T11)  [unwired: 10 in, 1 out]
        n125 = case shown="\"meTEC_CH1_Object Target Temperature (ID 3000 / 50012) [°C]\"" w238 {
          tunnel: w241 -> [w242 w256 w284 w292 w300 w310 w320 w328 w336 w345 w364 w382 w390 w398 w406 w411 w417]
          tunnel: [w242 w254 w284 w291 w299 w309 w319 w327 w335 w344 w363 w381 w389 w397 w405 w409 w415] -> w240
          tunnel: w239 -> [w244 w258 w286 w294 w302 w312 w322 w330 w338 w347 w366 w384 w392 w400 w408 w414 w420]
          tunnel: w237 -> [_ w255 _ w290 w298 w306 w314 w326 w334 w342 w361 w380 w388 w396 w404 w412 w418]
          tunnel: w236 -> [_ w248 _ _ _ _ _ _ _ _ _ _ _ _ _ _ _]
          frame "Blank", Default {
            n126 = property class="Str"(reference=w244, "Value"="To do...") -> ()  [unwired: 1 in, 2 out]
          }
          frame "meTEC_Reset Device" {
            n127 = flat-sequence {
              tunnel: w255 -> [w261]
              tunnel: w256 -> [w262]
              tunnel: [w262] -> w253
              tunnel: [w261] -> w252
              tunnel: w248 -> [w259]
              tunnel: [w259] -> w247
              tunnel: w253 -> [w270]
              tunnel: w252 -> [w269]
              tunnel: [w268] -> w251
              tunnel: [w267] -> w250
              tunnel: w247 -> [w265]
              tunnel: [w265] -> w245
              tunnel: w251 -> [w276]
              tunnel: w250 -> [w274]
              tunnel: [w275] -> w249
              tunnel: [w271] -> w246
              tunnel: w245 -> [w271]
              tunnel: [w279] -> w254
              tunnel: w249 -> [w280]
              tunnel: w246 -> [w278]
              frame #0 {
                # "Stop monitoring loop and wait\nuntil it actually stopped"
                n128 = while {
                  stop <- w264 continue-if-true
                  n129 = global read "Global_TEC Monitor Loop_Status.vi" "Monitoring Active?"() -> (w264:bool)
                  n130 = Wait Until Next ms Multiple(millisecond multiple=u32 50) -> ()  [unwired: 1 out]
                }
                n131 = global write "Global_TEC Monitor Loop_Status.vi" "Reset"(TRUE ("Reset")) -> ()
              }
              frame #1 {
                # "Reset TEC"
                n132 = Unbundle By Name(w269) -> ("PVs.TEC Configuration"=w267:T12)
                n133 = global write "Global_Initialized.vi" "Initialized_Step1?"(FALSE ("Initialized_Step1?")) -> ()
                n134 = call "meTEC_Reset Device.vi"("error in (no error)"=w270, "TEC Configuration_IN"=w267) -> ("error out"=w268:errorcluster)  [unwired: 7 in, 2 out]
              }
              frame #2 {
                # "Close COM port"
                n135 = Unbundle By Name(w274) -> ("VISA resource name"=w273:refnum<visa-resource-name>)
                n136 = Wait (ms)(milliseconds to wait=u32 200) -> ()  [unwired: 1 out]
                n137 = VISA Close(VISA resource name=w273, error in (no error)=w276) -> (error out=w275:errorcluster)
              }
              frame #3 {
                w277 = T8[] [{"Parameter"="", "Variant"=variant, "Main Loop States"=enum."Initialize"}, {"Parameter"="", "Variant"=variant, "Main Loop States"=enum."Idle"}]  # Elements to enqueue (Array) for initialization
                # "Trigger initialization\nprocess"
                n138 = global write "Global_TEC Monitor Loop_Status.vi" "Reset"(FALSE ("Reset")) -> ()
                n139 = call "Multiple Element Enqueue - Main Loop.vi"("error in (no error)"=w280, "Elements to enqueue (Array)"=w277, "Queue In"=w278) -> ("error out"=w279:errorcluster)  [unwired: 7 in, 1 out]
              }
            }
            n140 = property class="Str"(reference=w258, "Value"="Resetting TEC...") -> ()  [unwired: 1 in, 2 out]
          }
          frame "Return Front Panel Controls to TEC Reset State" {
            w282 = 0 items=["Parameter ID 3000 (Reset State)", "Parameter ID 50012"]
            w283 = 0 items=["Disabled (Reset State)", "Enabled"]
            n141 = property on="meTEC_CH1_Live Enable (ID 50000)" class="Ring (strict)"("Value"=w283) -> ()  [unwired: 2 in, 2 out]
            n142 = property on="meTEC_CH2_Live Enable (ID 50000)" class="Ring (strict)"("Value"=w283) -> ()  [unwired: 2 in, 2 out]
            n143 = property on="meTEC_CH1_Object Target Temp. Source Selection (ID 50011)" class="Ring (strict)"("Value"=w282) -> ()  [unwired: 2 in, 2 out]
            n144 = property on="meTEC_CH2_Object Target Temp. Source Selection (ID 50011)" class="Ring (strict)"("Value"=w282) -> ()  [unwired: 2 in, 2 out]
            n145 = property class="Str"(reference=w286, "Value"="Returning Front Panel Controls to TEC Reset State..") -> ()  [unwired: 1 in, 2 out]
          }
          frame "meTEC_CH1_Input Selection (ID 2000)" {
            n146 = Unbundle By Name(w290) -> ("PVs.TEC Configuration"=w289:T12)
            n147 = property class="Str"(reference=w294, "Value"="Selecting TEC Input...") -> ()  [unwired: 1 in, 2 out]
            n148 = call "meTEC_Set_ID 2000_Input Selection.vi"("Instance (1)"=u8 1, "error in (no error)"=w292, "TEC Configuration_IN"=w289, "Input Selection (ID 2000)"="meTEC_CH1_Input Selection (ID 2000)") -> ("error out"=w291:errorcluster)  [unwired: 5 in, 2 out]
          }
          frame "meTEC_CH2_Input Selection (ID 2000)" {
            n149 = Unbundle By Name(w298) -> ("PVs.TEC Configuration"=w297:T12)
            n150 = property class="Str"(reference=w302, "Value"="Selecting TEC Input...") -> ()  [unwired: 1 in, 2 out]
            n151 = call "meTEC_Set_ID 2000_Input Selection.vi"("Instance (1)"=u8 2, "error in (no error)"=w300, "TEC Configuration_IN"=w297, "Input Selection (ID 2000)"="meTEC_CH2_Input Selection (ID 2000)") -> ("error out"=w299:errorcluster)  [unwired: 5 in, 2 out]
          }
          frame "meTEC_CH1_Object Target Temp. Source Selection (ID 50011)" {
            n152 = Unbundle By Name(w306) -> ("PVs.TEC Configuration"=w308:T12)
            n153 = property class="Str"(reference=w312, "Value"="Selecting TEC Object Target Temp. Source...") -> ()  [unwired: 1 in, 2 out]
            n154 = call "meTEC_Set_ID 50011_Object Target Temperature Source Selection.vi"("Instance (1)"=u8 1 ("Instance (0)"), "error in (no error)"=w310, "TEC Configuration_IN"=w308, "Object Target Temperature Source Selection (ID 50011)"="meTEC_CH1_Object Target Temp. Source Selection (ID 50011)") -> ("error out"=w309:errorcluster)  [unwired: 5 in, 2 out]
            n155 = Bundle By Name(cluster=w306, "PVs.Object Target Temperature Source_CH1"="meTEC_CH1_Object Target Temp. Source Selection (ID 50011)") -> (w305:T11)
            n156 = call "FGV_TE Controller.vi"("Operation (Read)"=FGV_Operations."Write", "FGV_TEC_IN"=w305) -> ()  [unwired: 8 in, 2 out]
          }
          frame "meTEC_CH2_Object Target Temp. Source Selection (ID 50011)" {
            n157 = Unbundle By Name(w314) -> ("PVs.TEC Configuration"=w318:T12)
            n158 = property class="Str"(reference=w322, "Value"="Selecting TEC Object Target Temp. Source...") -> ()  [unwired: 1 in, 2 out]
            n159 = call "meTEC_Set_ID 50011_Object Target Temperature Source Selection.vi"("Instance (1)"=u8 2 ("Instance (0)"), "error in (no error)"=w320, "TEC Configuration_IN"=w318, "Object Target Temperature Source Selection (ID 50011)"="meTEC_CH2_Object Target Temp. Source Selection (ID 50011)") -> ("error out"=w319:errorcluster)  [unwired: 5 in, 2 out]
            n160 = Bundle By Name(cluster=w314, "PVs.Object Target Temperature Source_CH2"="meTEC_CH2_Object Target Temp. Source Selection (ID 50011)") -> (w315:T11)
            n161 = call "FGV_TE Controller.vi"("Operation (Read)"=FGV_Operations."Write", "FGV_TEC_IN"=w315) -> ()  [unwired: 8 in, 2 out]
          }
          frame "meTEC_CH1_Live Enable (ID 50000)" {
            n162 = Unbundle By Name(w326) -> ("PVs.TEC Configuration"=w325:T12)
            n163 = property class="Str"(reference=w330, "Value"="Enable / Disable Output...") -> ()  [unwired: 1 in, 2 out]
            n164 = call "meTEC_Set_ID 50000_Live Enable.vi"("Instance (1)"=u8 1 ("Instance (0)"), "error in (no error)"=w328, "TEC Configuration_IN"=w325, "Live Enable (ID 50000)"="meTEC_CH1_Live Enable (ID 50000)") -> ("error out"=w327:errorcluster)  [unwired: 5 in, 2 out]
          }
          frame "meTEC_CH2_Live Enable (ID 50000)" {
            n165 = Unbundle By Name(w334) -> ("PVs.TEC Configuration"=w333:T12)
            n166 = property class="Str"(reference=w338, "Value"="Enable / Disable Output...") -> ()  [unwired: 1 in, 2 out]
            n167 = call "meTEC_Set_ID 50000_Live Enable.vi"("Instance (1)"=u8 2 ("Instance (0)"), "error in (no error)"=w336, "TEC Configuration_IN"=w333, "Live Enable (ID 50000)"="meTEC_CH2_Live Enable (ID 50000)") -> ("error out"=w335:errorcluster)  [unwired: 5 in, 2 out]
          }
          frame "meTEC_CH1_Object Target Temperature (ID 3000 / 50012) [°C]" {
            # "0: ID 3000\n1: ID 50012"
            n168 = Unbundle By Name(w342) -> ("PVs.TEC Configuration"=w341:T12, "PVs.Object Target Temperature Source_CH1"=w339:u8)
            n169 = case shown="0, Default" w339 {
              tunnel: w345 -> [w352 w357]
              tunnel: [w351 w356] -> w344
              tunnel: "meTEC_CH1_Object Target Temperature (ID 3000 / 50012) [°C]" -> [w350 w355]
              tunnel: w341 -> [w349 w354]
              tunnel: u8 1 ("Instance") -> [w348 w353]
              frame 0, Default {
                n170 = call "meTEC_Set_ID 3000_Object Target Temperature.vi"("Instance (1)"=w348, "error in (no error)"=w352, "TEC Configuration_IN"=w349, "Object Target Temperature [°C]"=w350) -> ("error out"=w351:errorcluster)  [unwired: 5 in, 2 out]
              }
              frame 1 {
                n171 = call "meTEC_Set_ID 50012_Object Target Temperature.vi"("Instance (1)"=w353, "error in (no error)"=w357, "TEC Configuration_IN"=w354, "Object Target Temperature [°C]"=w355) -> ("error out"=w356:errorcluster)  [unwired: 5 in, 2 out]
              }
            }
            n172 = property class="Str"(reference=w347, "Value"="Setting TEC Object Target Temperature...") -> ()  [unwired: 1 in, 2 out]
          }
          frame "meTEC_CH2_Object Target Temperature (ID 3000 / 50012) [°C]" {
            # "0: ID 3000\n1: ID 50012"
            n173 = Unbundle By Name(w361) -> ("PVs.TEC Configuration"=w360:T12, "PVs.Object Target Temperature Source_CH2"=w358:u8)
            n174 = case shown="0, Default" w358 {
              tunnel: w364 -> [w371 w376]
              tunnel: [w370 w375] -> w363
              tunnel: "meTEC_CH2_Object Target Temperature (ID 3000 / 50012) [°C]" -> [w369 w374]
              tunnel: w360 -> [w368 w373]
              tunnel: u8 2 ("Instance") -> [w367 w372]
              frame 0, Default {
                n175 = call "meTEC_Set_ID 3000_Object Target Temperature.vi"("Instance (1)"=w367, "error in (no error)"=w371, "TEC Configuration_IN"=w368, "Object Target Temperature [°C]"=w369) -> ("error out"=w370:errorcluster)  [unwired: 5 in, 2 out]
              }
              frame 1 {
                n176 = call "meTEC_Set_ID 50012_Object Target Temperature.vi"("Instance (1)"=w372, "error in (no error)"=w376, "TEC Configuration_IN"=w373, "Object Target Temperature [°C]"=w374) -> ("error out"=w375:errorcluster)  [unwired: 5 in, 2 out]
              }
            }
            n177 = property class="Str"(reference=w366, "Value"="Setting TEC Object Target Temperature...") -> ()  [unwired: 1 in, 2 out]
          }
          frame "meTEC_CH1_Live Set Current (ID 50001) [A]" {
            n178 = Unbundle By Name(w380) -> ("PVs.TEC Configuration"=w379:T12)
            n179 = property class="Str"(reference=w384, "Value"="Setting TEC Live Set Current...") -> ()  [unwired: 1 in, 2 out]
            n180 = call "meTEC_Set_ID 50001_Live Set Current.vi"("Instance (1)"=u8 1 ("Instance"), "error in (no error)"=w382, "TEC Configuration_IN"=w379, "Live Current [A]"="meTEC_CH1_Live Set Current (ID 50001) [A]") -> ("error out"=w381:errorcluster)  [unwired: 5 in, 2 out]
          }
          frame "meTEC_CH2_Live Set Current (ID 50001) [A]" {
            n181 = Unbundle By Name(w388) -> ("PVs.TEC Configuration"=w387:T12)
            n182 = property class="Str"(reference=w392, "Value"="Setting TEC Live Set Current...") -> ()  [unwired: 1 in, 2 out]
            n183 = call "meTEC_Set_ID 50001_Live Set Current.vi"("Instance (1)"=u8 2 ("Instance"), "error in (no error)"=w390, "TEC Configuration_IN"=w387, "Live Current [A]"="meTEC_CH2_Live Set Current (ID 50001) [A]") -> ("error out"=w389:errorcluster)  [unwired: 5 in, 2 out]
          }
          frame "meTEC_CH1_Live Set Voltage (ID 50002) [V]" {
            n184 = Unbundle By Name(w396) -> ("PVs.TEC Configuration"=w395:T12)
            n185 = property class="Str"(reference=w400, "Value"="Setting TEC Live Set Voltage...") -> ()  [unwired: 1 in, 2 out]
            n186 = call "meTEC_Set_ID 50002_Live Set Voltage.vi"("Instance (1)"=u8 1 ("Instance"), "error in (no error)"=w398, "TEC Configuration_IN"=w395, "Live Set Voltage [V]"="meTEC_CH1_Live Set Voltage (ID 50002) [V]") -> ("error out"=w397:errorcluster)  [unwired: 5 in, 2 out]
          }
          frame "meTEC_CH2_Live Set Voltage (ID 50002) [V]" {
            n187 = Unbundle By Name(w404) -> ("PVs.TEC Configuration"=w403:T12)
            n188 = property class="Str"(reference=w408, "Value"="Setting TEC Live Set Voltage...") -> ()  [unwired: 1 in, 2 out]
            n189 = call "meTEC_Set_ID 50002_Live Set Voltage.vi"("Instance (1)"=u8 2 ("Instance"), "error in (no error)"=w406, "TEC Configuration_IN"=w403, "Live Set Voltage [V]"="meTEC_CH2_Live Set Voltage (ID 50002) [V]") -> ("error out"=w405:errorcluster)  [unwired: 5 in, 2 out]
          }
          frame "meTEC_Error Test 1_ID100_Device Type" {
            n190 = Unbundle By Name(w412) -> ("PVs.TEC Configuration"=w410:T12)
            n191 = property class="Str"(reference=w414, "Value"="Testing Error 1...") -> ()  [unwired: 1 in, 2 out]
            n192 = call "meTEC_Error Test_Read_ID 100_Device Type.vi"("error in (no error)"=w411, "TEC Configuration_IN"=w410) -> ("error out"=w409:errorcluster)  [unwired: 6 in, 3 out]
          }
          frame "meTEC_Perform Test" {
            # "Here you can place any VI for testing \nand execute it by pressing the \"Perform Test\" button\non the \"Error History\" tab."
            n193 = Unbundle By Name(w418) -> ("PVs.TEC Configuration"=w416:T12)
            n194 = property class="Str"(reference=w420, "Value"="Testing...") -> ()  [unwired: 1 in, 2 out]
            n195 = call "meTEC_Limit Read_ID 3000_Object Target Temperature.vi"("error in (no error)"=w417, "TEC Configuration_IN"=w416) -> ("error out"=w415:errorcluster)  [unwired: 6 in, 3 out]
          }
        }
      }
    }
  }
  n196 = while "Event Handling Loop" {
    tunnel: w2 -> [w423]
    tunnel: w5 -> [w422]
    stop <- w424 stop-if-true
    # ">> Error Queue >>"
    # ">> Main Queue >>"
    n197 = event shown="[5] \"meTEC_CH1_Object Target Temperature (ID 3000 / 50012) [°C]\", \"meTEC_CH2_Object Target Temperature (ID 3000 / 50012) [°C]\": Value Change" {
      selector: _ -> [_ _ _ _ _ _ _ _ _ _ _ _]
      dyn-events: _ -> [_ _ _ _ _ _ _ _ _ _ _ _]
      timeout: _ -> [_ _ _ _ _ _ _ _ _ _ _ _]
      tunnel: [w432 w439 w442 w448 w454 w460 w466 w472 w478 w485 w488 w494] -> w425
      tunnel: [w427 w434 _ _ _ _ _ _ _ _ _ _] -> w424
      tunnel: [errorcluster {"status"=FALSE, "code"=5000, "source"=""} ("element") errorcluster {"status"=FALSE, "code"=5000, "source"=""} ("element") _ _ _ _ _ _ _ _ _ _] -> w421
      event Application Instance Close? {
        n198 = event-data() -> ()  [unwired: 1 in, 4 out]
        n199 = Two Button Dialog(message="Are you sure you want to quit?") -> (T button?=w427:bool)  [unwired: 2 in]
        n200 = Select(t=T8[] [{"Parameter"="", "Variant"=variant, "Main Loop States"=enum."Shutdown"}] ("Elements to enqueue (Array)"), s=w427, f=T8[] [{"Parameter"="", "Variant"=variant, "Main Loop States"=enum."Idle"}] ("Elements to enqueue (Array)")) -> (s? t:f=w432:T8[])
        n201 = global write "Global_Quit.vi" "Quit"(w427) -> ()
        n202 = event-data("Discard?"=TRUE) -> ()  [unwired: 2 in, 1 out]
      }
      event Panel Close? {
        n203 = event-data() -> ()  [unwired: 1 in, 3 out]
        n204 = Two Button Dialog(message="Are you sure you want to quit?") -> (T button?=w434:bool)  [unwired: 2 in]
        n205 = Select(t=T8[] [{"Parameter"="", "Variant"=variant, "Main Loop States"=enum."Shutdown"}] ("Elements to enqueue (Array)"), s=w434, f=T8[] [{"Parameter"="", "Variant"=variant, "Main Loop States"=enum."Idle"}] ("Elements to enqueue (Array)")) -> (s? t:f=w439:T8[])
        n206 = global write "Global_Quit.vi" "Quit"(w434) -> ()
        n207 = event-data("Discard?"=TRUE) -> ()  [unwired: 1 in, 1 out]
      }
      event Value Change {
        n208 = event-data() -> ("CtlRef"=w441:refnum<vi>)  [unwired: 1 in, 4 out]
        n209 = property class="Ring (strict)"(reference=w441) -> ("Label.Text"=w444:string)  [unwired: 1 in, 2 out]
        n210 = Bundle By Name(cluster=T8 {"Parameter"="", "Variant"=variant, "Main Loop States"=enum."TE Controller"} ("Main Loop Queue Data"), "Parameter"=w444) -> (w443:T8)
        n211 = Build Array(w443, T8 {"Parameter"="", "Variant"=variant, "Main Loop States"=enum."Idle"} ("Main Loop Queue Data")) -> (w442:T8[])
      }
      event Value Change {
        n212 = event-data() -> ("CtlRef"=w447:refnum<vi>)  [unwired: 1 in, 4 out]
        n213 = property class="Ring (strict)"(reference=w447) -> ("Label.Text"=w450:string)  [unwired: 1 in, 2 out]
        n214 = Bundle By Name(cluster=T8 {"Parameter"="", "Variant"=variant, "Main Loop States"=enum."TE Controller"} ("Main Loop Queue Data"), "Parameter"=w450) -> (w449:T8)
        n215 = Build Array(w449, T8 {"Parameter"="", "Variant"=variant, "Main Loop States"=enum."Idle"} ("Main Loop Queue Data")) -> (w448:T8[])
      }
      event Value Change {
        n216 = event-data() -> ("CtlRef"=w453:refnum<vi>)  [unwired: 1 in, 4 out]
        n217 = property class="Ring (strict)"(reference=w453) -> ("Label.Text"=w456:string)  [unwired: 1 in, 2 out]
        n218 = Bundle By Name(cluster=T8 {"Parameter"="", "Variant"=variant, "Main Loop States"=enum."TE Controller"} ("Main Loop Queue Data"), "Parameter"=w456) -> (w455:T8)
        n219 = Build Array(w455, T8 {"Parameter"="", "Variant"=variant, "Main Loop States"=enum."Idle"} ("Main Loop Queue Data")) -> (w454:T8[])
      }
      event "meTEC_CH1_Object Target Temperature (ID 3000 / 50012) [°C]", "meTEC_CH2_Object Target Temperature (ID 3000 / 50012) [°C]": Value Change {
        n220 = event-data() -> ("CtlRef"=w459:refnum<vi>)  [unwired: 1 in, 4 out]
        n221 = property class="DigNum (strict)"(reference=w459) -> ("Label.Text"=w462:string)  [unwired: 1 in, 2 out]
        n222 = Bundle By Name(cluster=T8 {"Parameter"="", "Variant"=variant, "Main Loop States"=enum."TE Controller"} ("Main Loop Queue Data"), "Parameter"=w462) -> (w461:T8)
        n223 = Build Array(w461, T8 {"Parameter"="", "Variant"=variant, "Main Loop States"=enum."Idle"} ("Main Loop Queue Data")) -> (w460:T8[])
      }
      event "meTEC_CH1_Live Set Current (ID 50001) [A]", "meTEC_CH2_Live Set Current (ID 50001) [A]": Value Change {
        n224 = event-data() -> ("CtlRef"=w465:refnum<vi>)  [unwired: 1 in, 4 out]
        n225 = property class="DigNum (strict)"(reference=w465) -> ("Label.Text"=w468:string)  [unwired: 1 in, 2 out]
        n226 = Bundle By Name(cluster=T8 {"Parameter"="", "Variant"=variant, "Main Loop States"=enum."TE Controller"} ("Main Loop Queue Data"), "Parameter"=w468) -> (w467:T8)
        n227 = Build Array(w467, T8 {"Parameter"="", "Variant"=variant, "Main Loop States"=enum."Idle"} ("Main Loop Queue Data")) -> (w466:T8[])
      }
      event "meTEC_CH1_Live Set Voltage (ID 50002) [V]", "meTEC_CH2_Live Set Voltage (ID 50002) [V]": Value Change {
        n228 = event-data() -> ("CtlRef"=w471:refnum<vi>)  [unwired: 1 in, 4 out]
        n229 = property class="DigNum (strict)"(reference=w471) -> ("Label.Text"=w474:string)  [unwired: 1 in, 2 out]
        n230 = Bundle By Name(cluster=T8 {"Parameter"="", "Variant"=variant, "Main Loop States"=enum."TE Controller"} ("Main Loop Queue Data"), "Parameter"=w474) -> (w473:T8)
        n231 = Build Array(w473, T8 {"Parameter"="", "Variant"=variant, "Main Loop States"=enum."Idle"} ("Main Loop Queue Data")) -> (w472:T8[])
      }
      event "meTEC_Reset Device": Value Change {
        n232 = event-data() -> ("CtlRef"=w477:refnum<vi>)  [unwired: 1 in, 4 out]
        n233 = property class="Bool"(reference=w477) -> ("Label.Text"=w480:string)  [unwired: 1 in, 2 out]
        n234 = Bundle By Name(cluster=T8 {"Parameter"="", "Variant"=variant, "Main Loop States"=enum."TE Controller"} ("Main Loop Queue Data"), "Parameter"=w480) -> (w479:T8)
        n235 = Build Array(w479, T8 {"Parameter"="Return Front Panel Controls to TEC Reset State", "Variant"=variant, "Main Loop States"=enum."TE Controller"} ("Main Loop Queue Data")) -> (w478:T8[])
      }
      event "meTEC_Initialize Device": Value Change {
        # "Reset boolean control to\ninitial value"
        n236 = event-data() -> ()  [unwired: 1 in, 1 out]
        n237 = local write "meTEC_Initialize Device"(FALSE ("meTEC_Initialize Device")) -> ()
        n238 = Build Array(T8 {"Parameter"="", "Variant"=variant, "Main Loop States"=enum."Initialize"} ("Main Loop Queue Data"), T8 {"Parameter"="", "Variant"=variant, "Main Loop States"=enum."Idle"} ("Main Loop Queue Data")) -> (w485:T8[])
      }
      event "meTEC_Error Test 1_ID100_Device Type": Value Change {
        n239 = event-data() -> ("CtlRef"=w487:refnum<vi>)  [unwired: 1 in, 4 out]
        n240 = property class="Bool"(reference=w487) -> ("Label.Text"=w490:string)  [unwired: 1 in, 2 out]
        n241 = Bundle By Name(cluster=T8 {"Parameter"="", "Variant"=variant, "Main Loop States"=enum."TE Controller"} ("Main Loop Queue Data"), "Parameter"=w490) -> (w489:T8)
        n242 = Build Array(w489, T8 {"Parameter"="", "Variant"=variant, "Main Loop States"=enum."Idle"} ("Main Loop Queue Data")) -> (w488:T8[])
      }
      event "meTEC_Perform Test": Value Change {
        n243 = event-data() -> ("CtlRef"=w493:refnum<vi>)  [unwired: 1 in, 4 out]
        n244 = property class="Bool"(reference=w493) -> ("Label.Text"=w496:string)  [unwired: 1 in, 2 out]
        n245 = Bundle By Name(cluster=T8 {"Parameter"="", "Variant"=variant, "Main Loop States"=enum."TE Controller"} ("Main Loop Queue Data"), "Parameter"=w496) -> (w495:T8)
        n246 = Build Array(w495, T8 {"Parameter"="", "Variant"=variant, "Main Loop States"=enum."Idle"} ("Main Loop Queue Data")) -> (w494:T8[])
      }
    }
    n247 = call "Multiple Element Enqueue - Main Loop.vi"("Elements to enqueue (Array)"=w425, "Queue In"=w423) -> ()  [unwired: 8 in, 2 out]
    n248 = call "Error Queue - Enqueue Element.vi"("error in (no error)"=w421, "Error Queue IN"=w422) -> ()  [unwired: 9 in, 1 out]
  }
  n249 = Merge Errors(w23, w22, w13) -> (w21:errorcluster)
  n250 = call <vilib>:"General Error Handler.vi"("error in (no error)"=w21) -> ("error out"=w16:errorcluster)  [unwired: 10 in, 4 out]
  n251 = call "Clear All Errors.vi"("error in (no error)"=w16) -> ("error out"=w10:errorcluster)  [unwired: 1 in]
  n252 = property class="App"(error in=w10) -> ("App.Kind"=w29:T9)  [unwired: 1 in, 2 out]
  n253 = Equal?(x=w29, y=T9."Run Time System") -> (x = y?=w27:bool)
  n254 = Quit LabVIEW(quit? (T)=w27) -> ()
